vi "BuildOutline.vi"(8 "Setup":T1={"Scaling (pixels/mm)"=1.0, "Tool Diameter (inch)"=0.25, "Origin location"={"x (mm)"=10, "y (mm)"=300}, "Wood dim"={"width (inch)"=10.0, "height (inch)"=300.0}}, 11 "Bounds":T2) -> (1 "new picture":picture, 3 "outline box":cluster{dbl, dbl, dbl, dbl})   [LabVIEW 2023]
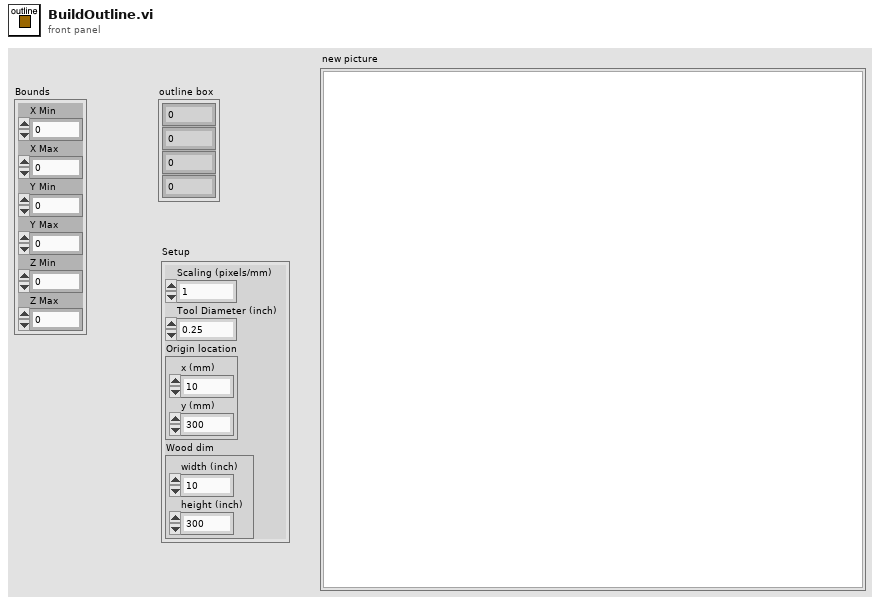
[diagram p1: front panel]
types:
  T1 = cluster{"Scaling (pixels/mm)":dbl, "Tool Diameter (inch)":dbl, "Origin location":cluster{"x (mm)":i16, "y (mm)":i16}, "Wood dim":cluster{"width (inch)":dbl, "height (inch)":dbl}}
  T2 = cluster{"X Min":dbl, "X Max":dbl, "Y Min":dbl, "Y Max":dbl, "Z Min":dbl, "Z Max":dbl}
  T3 = cluster{"left":i16, "top":i16, "right":i16, "bottom":i16}
  T4 = cluster{"x (mm)":i16, "y (mm)":i16, "x (mm)":i16, "y (mm)":i16}
  T5 = cluster{"left":dbl, "top":dbl, "right":dbl, "bottom":dbl}
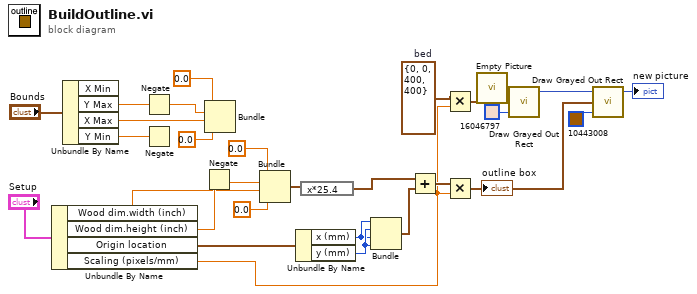
[diagram p0: block diagram]
diagram:
  w14 = T3 {"left"=0, "top"=0, "right"=400, "bottom"=400}  # bed
  n1 = Unbundle By Name("Setup") -> ("Wood dim.width (inch)"=w1:dbl, "Wood dim.height (inch)"=w5:dbl, "Origin location"=w17:cluster{"x (mm)":i16, "y (mm)":i16}, "Scaling (pixels/mm)"=w10:dbl)
  n2 = Unbundle By Name("Bounds") -> ("Y Max"=w23:dbl, "X Max"=w22:dbl, "Y Min"=w24:dbl)  [unwired: 1 out]
  n3 = Negate(x=w23) -> (-x=w29:dbl)
  n4 = Negate(x=w24) -> ()  [unwired: 1 out]
  n5 = Negate(x=w5) -> (-x=w2:dbl)
  n6 = Bundle(0.0, w29, "X Max"=w22, 0.0) -> ()  [unwired: 1 in, 1 out]
  n7 = Bundle(0.0, w2, "width (inch)"=w1, 0.0) -> (w4:cluster{dbl, dbl, "width (inch)":dbl, dbl})  [unwired: 1 in]
  n8 = Unbundle By Name(w17) -> ("x (mm)"=w25:i16, "y (mm)"=w26:i16)
  n9 = expression code="x*25.4"(w4) -> (w3:cluster{dbl, dbl, "width (inch)":dbl, dbl})
  n10 = Bundle("x (mm)"=w25, "y (mm)"=w26, "x (mm)"=w25, "y (mm)"=w26) -> (w27:T4)  [unwired: 1 in]
  n11 = Add(x=w3, y=w27) -> (x+y=w28:cluster{dbl, dbl, dbl, dbl})
  n12 = Multiply(x=w14, y=w10) -> (x*y=w13:T5)
  n13 = Multiply(x=w28, y=w10) -> (x*y=w9:cluster{dbl, dbl, dbl, dbl})
  "outline box" <- w9
  n14 = call "Empty Picture"() -> ("empty picture"=w16:picture)
  n15 = call <vilib>:"Draw Grayed Out Rect.vi"("color(black)"=u32 16046797, "rect"=w13, "picture"=w16) -> ("new picture"=w12:picture)  [unwired: 2 in]
  n16 = call <vilib>:"Draw Grayed Out Rect.vi"("color(black)"=u32 10443008, "rect"=w9, "picture"=w12) -> ("new picture"=→"new picture":picture)  [unwired: 2 in]
